vi "PAQmem_VerifyTimeRange.vi"(8 "error in (no error)":errorcluster, 9 "Time-End":timestamp, 10 "Time-Start":timestamp, 11 "PAQ-memory in":refnum<class "PAQ-memory.lvclass">) -> (0 "error out":errorcluster, 1 "TableName":string, 2 "All data in memory range":bool, 3 "PAQ-memory out":refnum<class "PAQ-memory.lvclass">)   [LabVIEW 2020, in "Sgraph_lib_V1.lvlib" / "PAQ-memory.lvclass"]
doc: "Check if the required memory to fetch is available within the available PAQ memory"
uses:
  PAQ-memory.lvclass
  PAQ-memory.lvclass/PAQ-memory.ctl
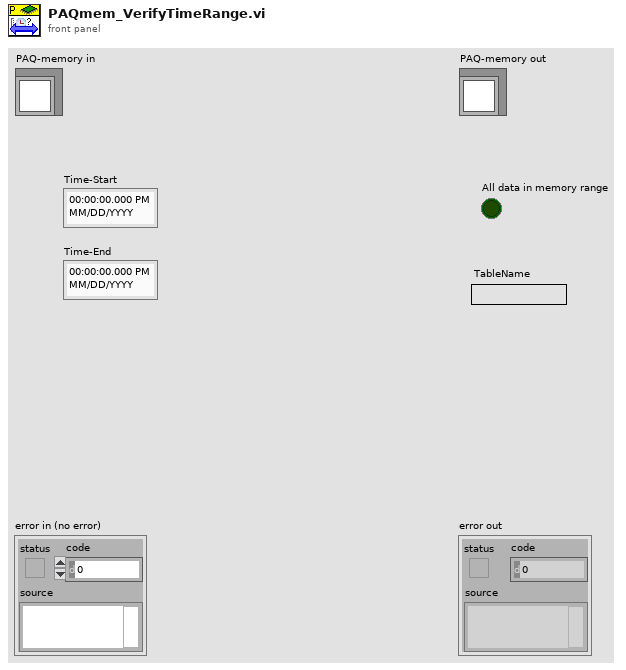
[diagram p1: front panel]
types:
  T1 = cluster{"Tmax":timestamp, "Tmin":timestamp, "IdxMax":i32, "IdxMin":i32}
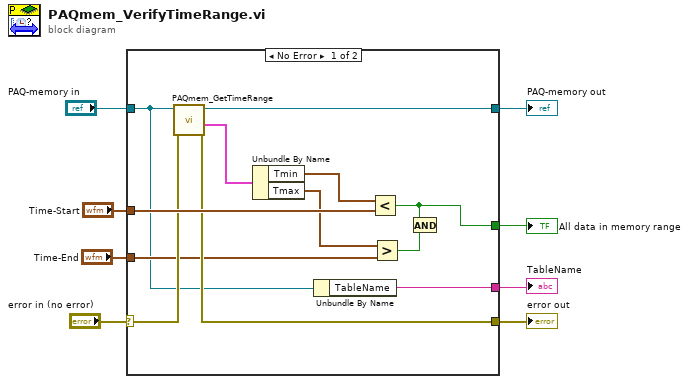
[diagram p0: block diagram]
diagram:
  n1 = case shown="No Error" "error in (no error)" {
    selector: "error in (no error)" -> [w15 w22]
    tunnel: [w14 w22] -> w7
    tunnel: [w20 w21] -> w5
    tunnel: "PAQ-memory in" -> [w10 w21]
    tunnel: "Time-Start" -> [w17 _]
    tunnel: "Time-End" -> [w12 _]
    tunnel: [w11 _] -> w2
    tunnel: [w9 _] -> w1
    frame No Error {
      n2 = call "PAQmem_GetTimeRange.vi"("error in (no error)"=w15, "PAQ-memory in"=w10) -> ("error out"=w14:errorcluster, "T_range"=w19:T1, "PAQ-memory out"=w20:refnum<class "PAQ-memory.lvclass">)  [unwired: 7 in]
      n3 = Unbundle By Name(w19) -> ("Tmin"=w18:timestamp, "Tmax"=w13:timestamp)
      n4 = Unbundle By Name(w10) -> ("TableName"=w9:string)
      n5 = Less?(x=w18, y=w17) -> (x < y?=w11:bool)
      n6 = Greater?(x=w13, y=w12) -> (0:w16:bool)
      n7 = And(x=w11, y=w16) -> ()  [unwired: 1 out]
    }
    frame Error {
    }
  }
  "error out" <- w7
  "PAQ-memory out" <- w5
  "All data in memory range" <- w2
  "TableName" <- w1
